vi "For Loop.vi"() -> ()   [LabVIEW 2023]
panel:
  in  "Numeric 2":i32
  out "Numeric":i32
  out "number (0 to 1)":dbl
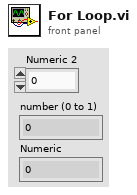
[diagram p1: front panel]
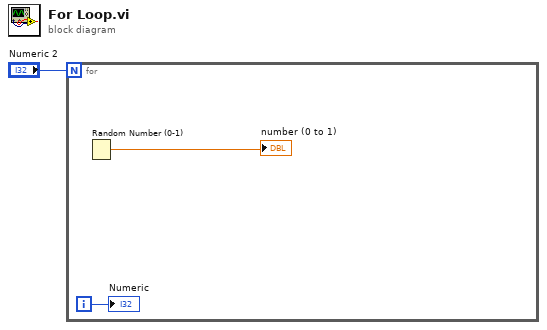
[diagram p0: block diagram]
diagram:
  n1 = for {
    N: "Numeric 2" -> [_]
    i -> [w2]
    n2 = Random Number (0-1)() -> (number: 0 to 1=→"number (0 to 1)":dbl)
    "Numeric" <- w2
  }
